vi "Prepare for external window.vi"(8 "error in (no error)":errorcluster, 11 "External Display":bool) -> (0 "error out":errorcluster)   [LabVIEW 2021, in "ImageStreamRendering.lvlib"]
uses:
  ImageStreamRendering.lvlib
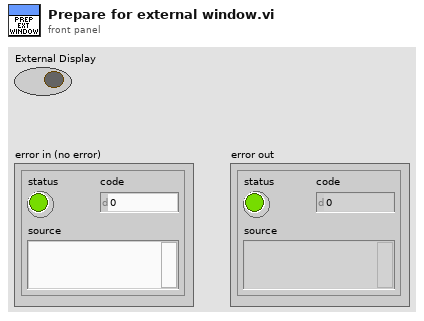
[diagram p1: front panel]
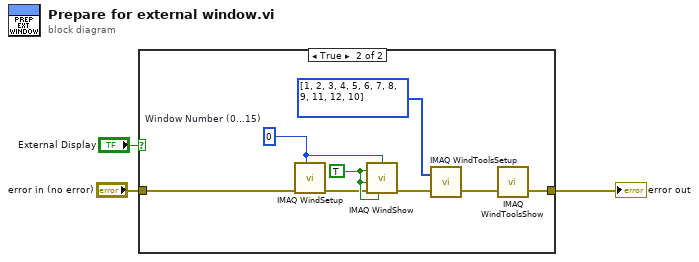
[diagram p0: block diagram]
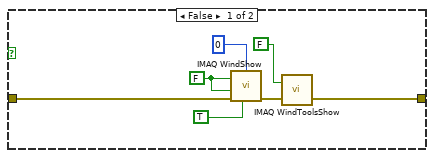
[diagram p2: hidden frame]
diagram:
  n1 = case shown="True" "External Display" {
    tunnel: "error in (no error)" -> [w5 w12]
    tunnel: [w4 w11] -> w2
    frame False {
      w9 = FALSE ("Hide/Show (Show)")
      n2 = call "IMAQ WindShow"("error in (no error)"=w5, "Bring To Front? (N)"=w9, "Get/Set Status? (Set)"=TRUE, "Hide/Show (Show)"=w9, "Window Number (0...15)"=0) -> ("error out"=w7:errorcluster)  [unwired: 1 in, 2 out]
      n3 = call "IMAQ WindToolsShow"("Hide/Show (Show)"=FALSE, "error in (no error)"=w7) -> ("error out"=w4:errorcluster)  [unwired: 3 in, 1 out]
    }
    frame True {
      w13 = 0  # Window Number (0...15)
      w17 = u32[] [1, 2, 3, 4, 5, 6, 7, 8, 9, 11, 12, 10] items=["No Selection", "Point", "Line", "Rectangle", "Oval", "Polygon", "Freehand Region", "Annulus", "Zoom", "Pan", "Broken Line", "Freehand Line", "Rotated Rectangle"] ("Tools")
      w18 = TRUE ("Bring To Front? (N)")
      n4 = call "IMAQ WindSetup"("Window Number (0...15)"=w13, "error in (no error)"=w12) -> ("error out"=w14:errorcluster)  [unwired: 9 in]
      n5 = call "IMAQ WindShow"("error in (no error)"=w14, "Bring To Front? (N)"=w18, "Get/Set Status? (Set)"=w18, "Hide/Show (Show)"=w18, "Window Number (0...15)"=w13) -> ("error out"=w16:errorcluster)  [unwired: 1 in, 2 out]
      n6 = call "IMAQ WindToolsSetup"("Tools"=w17, "error in (no error)"=w16) -> ("error out"=w15:errorcluster)  [unwired: 4 in]
      n7 = call "IMAQ WindToolsShow"("error in (no error)"=w15) -> ("error out"=w11:errorcluster)  [unwired: 4 in, 1 out]
    }
  }
  "error out" <- w2
